vi "ReadtextandwriteSql.vi"() -> ()   [LabVIEW 2019]
uses:
  <vilib>/addons/database/Auxilliary.llb/DB Tools Parameter Info.ctl
  <vilib>/addons/database/Auxilliary.llb/DB Tools DataTypes.ctl
  <vilib>/addons/database/Auxilliary.llb/DB Tools Parameter Dir.ctl
  <vilib>/addons/database/Connection.llb/DB Tools Open Connec (String).vi
  <vilib>/Utility/file.llb/Read Delimited Spreadsheet (string).vi
  <vilib>/addons/database/Auxilliary.llb/DB Tools Format Datetime String (Time Stamp).vi
  <vilib>/addons/database/Command.llb/Cmd Set Parameter Value (C).vi
  <vilib>/addons/database/Command.llb/Cmd Execute.vi
  <vilib>/addons/database/Recordset.llb/Rec Destroy - Command.vi
  <vilib>/addons/database/Command.llb/Cmd Delete.vi
  <vilib>/addons/database/NI_Database_API.lvlib
panel:
  out "spreadsheet string":string
  out "insert time":timestamp
  out "total time in opreation":dbl
  out "Program start time":timestamp
  out "size(s)":i32[](array[numeric])
  out "Current Number of file":i32
  out "Current record number":i32
  out "all rows 2":string[](array[string])
  out "all rows":string[][](array[string])
  out "Total  Content Read from file":i32
  out "Content of Current file":string
  out "Current File path":path
  out "No of text files in folder":dbl
  in  "Input for folder path":path
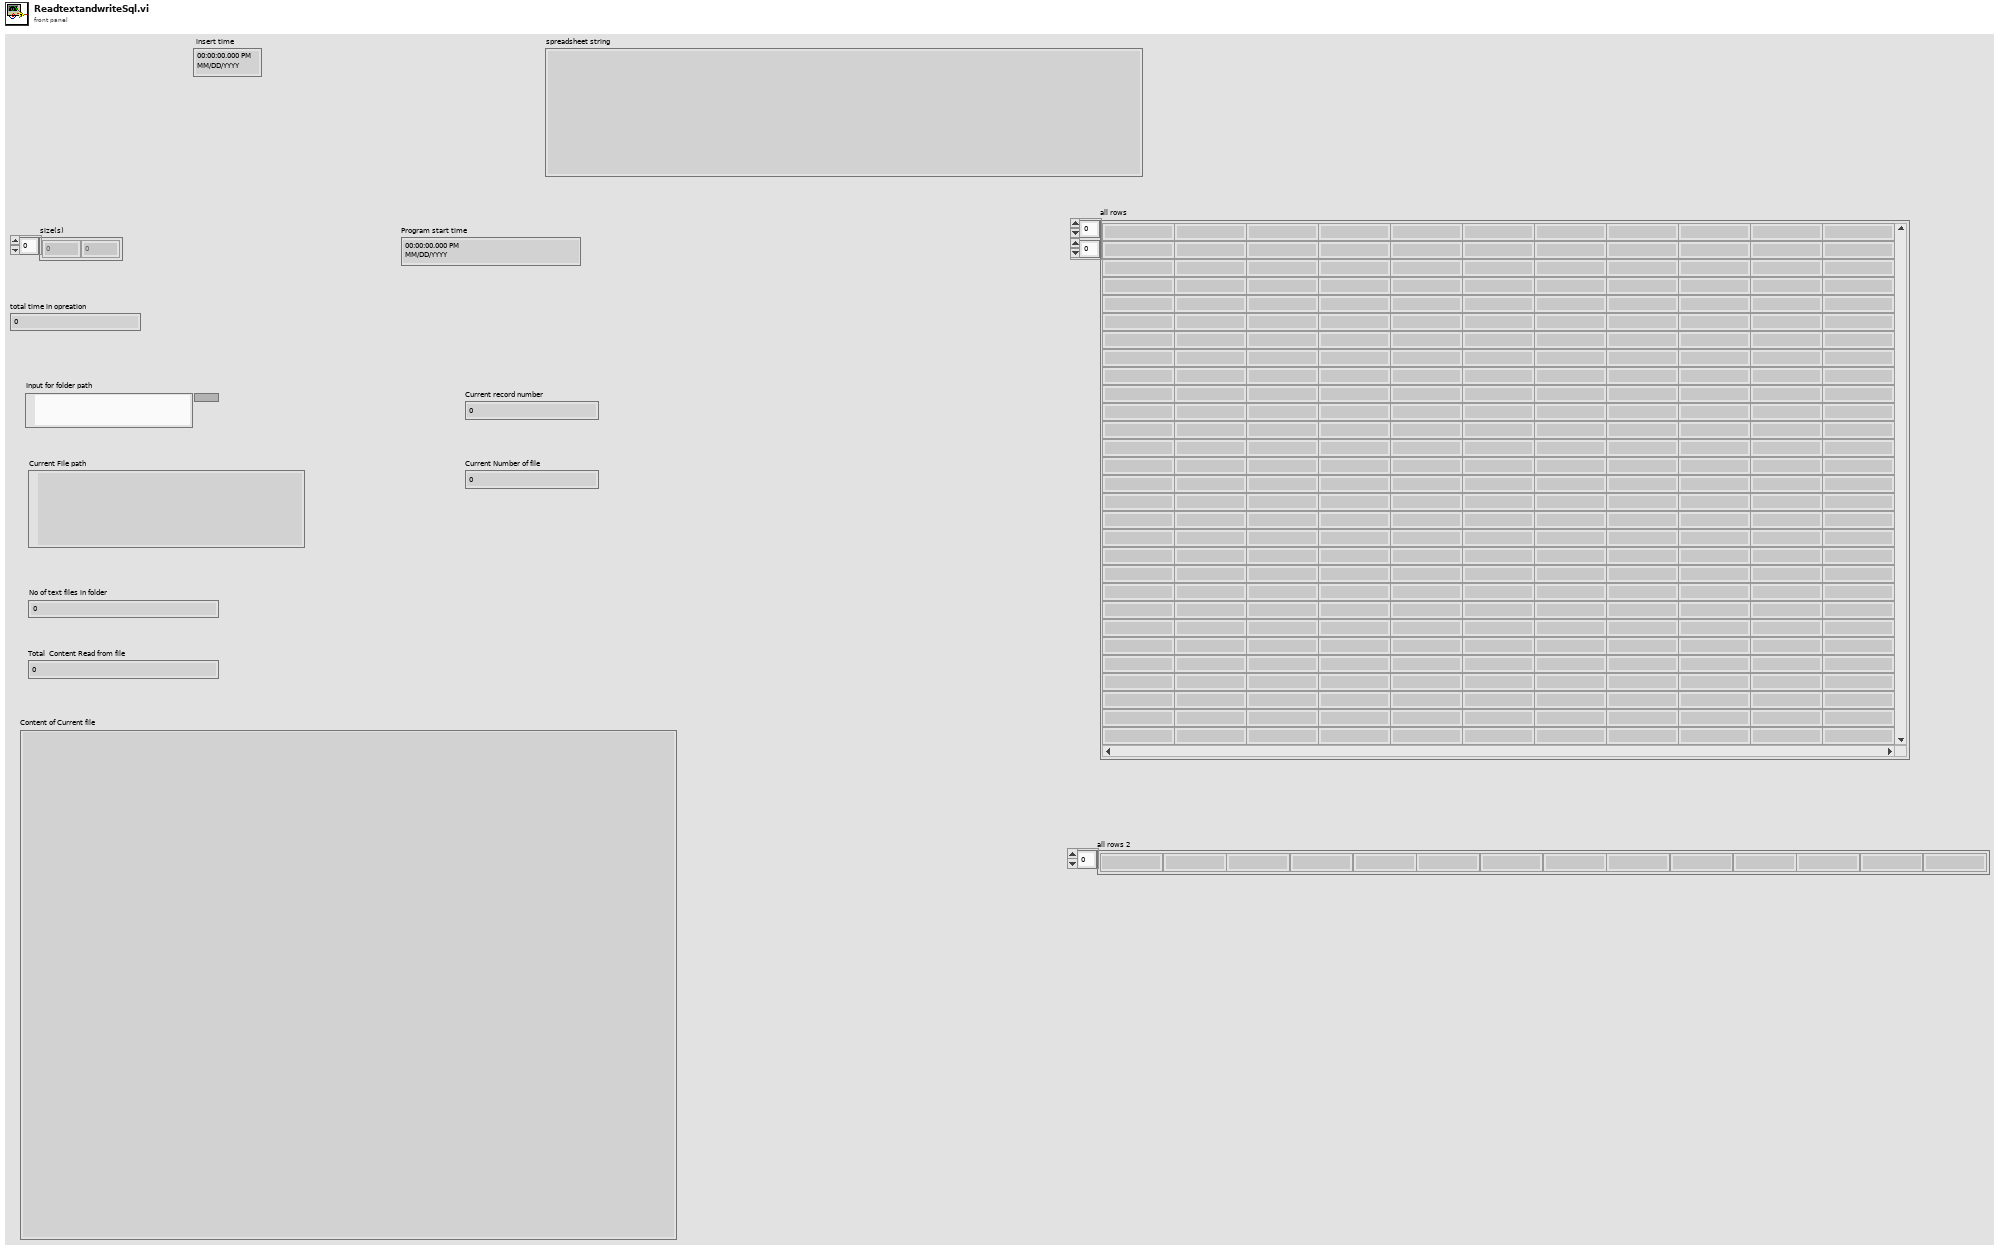
[diagram p1: front panel]
types:
  T1 = typedef "NI_Database_API.lvlib/DB Tools Parameter Info.ctl" = cluster{"parameter name":string, "type":T2, "direction":T3, "value":variant}
  T2 = typedef "NI_Database_API.lvlib/DB Tools DataTypes.ctl" = enum16{"String", "Long (I32)", "Single (SGL)", "Double (DBL)", "Date/Time", "Binary"}
  T3 = typedef "NI_Database_API.lvlib/DB Tools Parameter Dir.ctl" = enum32{"Input", "Output", "Input/Output", "Return Value"}
  T4 = typedef "NI_Database_API.lvlib/Conn ObjectReference.ctl" = refnum<k1>
  T5 = typedef "NI_Database_API.lvlib/Cmd ObjectReference.ctl" = refnum<k1>
  T6 = typedef "NI_Database_API.lvlib/Cmd-Rec Object Reference.ctl" = refnum<k1>
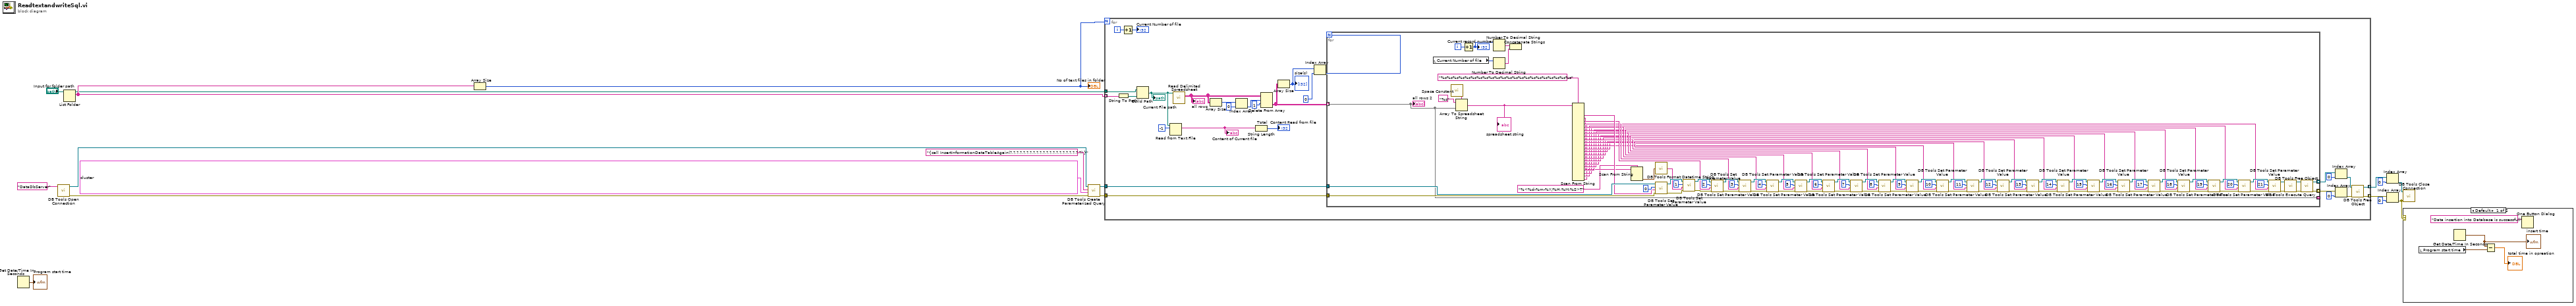
[diagram p0: block diagram]
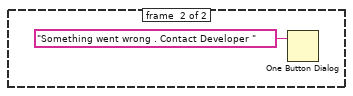
[diagram p2: hidden frame]
diagram:
  n1 = Get Date/Time In Seconds() -> (seconds since 1Jan1904=→"Program start time":timestamp)
  n2 = call-poly <vilib>:"DB Tools Open Connection.vi"("connection information"="DataDbServer") -> ("error out"=w13:errorcluster, "connection reference"=w12:T4)  [unwired: 7 in]
  n3 = List Folder(path="Input for folder path") -> (path out=w16:path, filenames=w17:string[])  [unwired: 3 in, 2 out]
  n4 = Array Size(array=w17) -> (size(s)=w14:i32)
  "No of text files in folder" <- w14
  n5 = call <vilib>:"DB Tools Create Parameterized Query.vi"("error in (no error)"=w13, "parameters"=T1[] [{"parameter name"="Start", "type"=enum."String", "direction"=enum."Input", "value"=variant}, {"parameter name"="DateTime", "type"=enum."Date/Time", "direction"=enum."Input", "value"=variant}, {"parameter name"="RollNo", "type"=enum."String", "direction"=enum."Input", "value"=variant}, {"parameter name"="Grade", "type"=enum."String", "direction"=enum."Input", "value"=variant}, {"parameter name"="BatchNO", "type"=enum."String", "direction"=enum."Input", "value"=variant}, {"parameter name"="product", "type"=enum."String", "direction"=enum."Input", "value"=variant}, {"parameter name"="OPName", "type"=enum."String", "direction"=enum."Input", "value"=variant}, {"parameter name"="shiftName", "type"=enum."String", "direction"=enum."Input", "value"=variant}, {"parameter name"="width", "type"=enum."String", "direction"=enum."Input", "value"=variant}, {"parameter name"="EWeight", "type"=enum."String", "direction"=enum."Input", "value"=variant}, {"parameter name"="TSetPoint", "type"=enum."String", "direction"=enum."Input", "value"=variant}, {"parameter name"="BSetPoint", "type"=enum."String", "direction"=enum."Input", "value"=variant}, {"parameter name"="col113", "type"=enum."String", "direction"=enum."Input", "value"=variant}, {"parameter name"="col14", "type"=enum."String", "direction"=enum."Input", "value"=variant}, {"parameter name"="col15", "type"=enum."String", "direction"=enum."Input", "value"=variant}, {"parameter name"="col16", "type"=enum."String", "direction"=enum."Input", "value"=variant}, {"parameter name"="col17", "type"=enum."String", "direction"=enum."Input", "value"=variant}, {"parameter name"="col18", "type"=enum."String", "direction"=enum."Input", "value"=variant}, {"parameter name"="col19", "type"=enum."String", "direction"=enum."Input", "value"=variant}, {"parameter name"="col20", "type"=enum."String", "direction"=enum."Input", "value"=variant}, {"parameter name"="col21", "type"=enum."String", "direction"=enum."Input", "value"=variant}, {"parameter name"="col22", "type"=enum."String", "direction"=enum."Input", "value"=variant}], "SQL query"="{call InsertInformationDataTableAgain(?,?,?,?,?,?,?,?,?,?,?,?,?,?,?,?,?,?,?,?,?,?) }", "connection reference"=w12) -> ("error out"=w8:errorcluster, "command reference"=w9:T5)  [unwired: 3 in, 1 out]
  n6 = for {
    N: w14 -> [_]
    tunnel: w17 -> [w46] mode=indexing
    tunnel: w16 -> [w45]
    tunnel: w9 -> [w34]
    tunnel: w8 -> [w33]
    tunnel: [w26] -> w7 mode=indexing
    tunnel: [w25] -> w5 mode=indexing
    i -> [w36]
    n7 = String To Path(string=w46) -> (path=w44:path)
    n8 = Increment(x=w36) -> (x+1=→"Current Number of file":i32)
    n9 = Build Path(base path=w45, name or relative path=w44) -> (appended path=w42:path)
    "Current File path" <- w42
    n10 = Read from Text File(file (use dialog)=w42, count=-1) -> (text=w41:string)  [unwired: 2 in, 3 out]
    "Content of Current file" <- w41
    n11 = call-poly <vilib>:"Read Delimited Spreadsheet.vi"("file path (dialog if empty)"=w42) -> ("all rows"=w20:string[][])  [unwired: 9 in, 5 out]
    "all rows" <- w20
    n12 = Array Size(array=w20) -> (size(s)=w24:i32[])
    n13 = Index Array(array=w24, index=0) -> (element=w22:i32)
    n14 = String Length(string=w41) -> (length=→"Total  Content Read from file":i32)
    n15 = Delete From Array(array=w20, length=w22, index (row)=1) -> (deleted portion=w19:string[][])  [unwired: 1 in, 1 out]
    n16 = Array Size(array=w19) -> (size(s)=w39:i32[])
    "size(s)" <- w39
    n17 = Index Array "Index Array"(array=w39, index=0) -> (element=w37:i32)
    n18 = for {
      N: w37 -> [_]
      tunnel: w19 -> [w51] mode=indexing
      tunnel: [w51] -> _ mode=indexing
      tunnel: w34 -> [w151]
      tunnel: w33 -> [w100]
      tunnel: [w78] -> w32 mode=indexing
      tunnel: [w77] -> w29 mode=indexing
      i -> [w103]
      n19 = local read "Current Number of file"() -> (w106:i32)
      n20 = call <vilib>:"Space Constant.vi"() -> ("String"=w50:string)
      n21 = Array To Spreadsheet String(delimiter (Tab)=w50, array=w51, 3:"%s" ("format string")) -> (spreadsheet string=w52:string)
      "spreadsheet string" <- w52
      n22 = Increment(x=w103) -> (x+1=w102:i32)
      "Current record number" <- w102
      n23 = Number To Decimal String(number=w102) -> (decimal integer string=w105:string)  [unwired: 1 in]
      n24 = Number To Decimal String(number=w106) -> (decimal integer string=w104:string)  [unwired: 1 in]
      n25 = Concatenate Strings(w105, w104) -> ()  [unwired: 1 out]
      n26 = Scan From String(format string="%s%s%s%s%s%s%s%s%s%s%s%s%s%s%s%s%s%s%s%s%s%s", input string=w52) -> (output 1=w74:string, output 2=w49:string, output 3=w73:string, output 4=w72:string, output 5=w71:string, output 6=w70:string, output 7=w69:string, output 8=w68:string, output 9=w67:string, output 10=w66:string, output 11=w65:string, output 12=w64:string, output 13=w63:string, output 14=w61:string, output 15=w60:string, output 16=w59:string, output 17=w58:string, output 18=w57:string, output 19=w56:string, output 20=w55:string, output 21=w54:string, output 22=w53:string)  [unwired: 24 in, 3 out]
      n27 = Scan From String(format string="%<%d-%m-%Y/%H:%M:%S>T", input string=w49) -> (output 1=w48:timestamp)  [unwired: 3 in, 3 out]
      n28 = call-poly <vilib>:"DB Tools Format Datetime String.vi"("time stamp"=w48) -> ("date/time string"=w75:string)
      n29 = call-poly <vilib>:"DB Tools Set Parameter Value.vi"("error in (no error)"=w100, "value"=w74, "parameter index"=0, "command reference"=w151) -> ("error out"=w101:errorcluster, "command reference out"=w149:T5)  [unwired: 4 in]
      n30 = call-poly <vilib>:"DB Tools Set Parameter Value.vi"("error in (no error)"=w101, "value"=w75, "parameter index"=1, "command reference"=w149) -> ("error out"=w147:errorcluster, "command reference out"=w146:T5)  [unwired: 4 in]
      n31 = call-poly <vilib>:"DB Tools Set Parameter Value.vi"("error in (no error)"=w147, "value"=w73, "parameter index"=2, "command reference"=w146) -> ("error out"=w143:errorcluster, "command reference out"=w144:T5)  [unwired: 4 in]
      n32 = call-poly <vilib>:"DB Tools Set Parameter Value.vi"("error in (no error)"=w143, "value"=w72, "parameter index"=3, "command reference"=w144) -> ("error out"=w98:errorcluster, "command reference out"=w141:T5)  [unwired: 4 in]
      n33 = call-poly <vilib>:"DB Tools Set Parameter Value.vi"("error in (no error)"=w98, "value"=w71, "parameter index"=4, "command reference"=w141) -> ("error out"=w139:errorcluster, "command reference out"=w140:T5)  [unwired: 4 in]
      n34 = call-poly <vilib>:"DB Tools Set Parameter Value.vi"("error in (no error)"=w139, "value"=w70, "parameter index"=5, "command reference"=w140) -> ("error out"=w136:errorcluster, "command reference out"=w137:T5)  [unwired: 4 in]
      n35 = call-poly <vilib>:"DB Tools Set Parameter Value.vi"("error in (no error)"=w136, "value"=w69, "parameter index"=6, "command reference"=w137) -> ("error out"=w133:errorcluster, "command reference out"=w134:T5)  [unwired: 4 in]
      n36 = call-poly <vilib>:"DB Tools Set Parameter Value.vi"("error in (no error)"=w133, "value"=w68, "parameter index"=7, "command reference"=w134) -> ("error out"=w130:errorcluster, "command reference out"=w131:T5)  [unwired: 4 in]
      n37 = call-poly <vilib>:"DB Tools Set Parameter Value.vi"("error in (no error)"=w130, "value"=w67, "parameter index"=8, "command reference"=w131) -> ("error out"=w127:errorcluster, "command reference out"=w128:T5)  [unwired: 4 in]
      n38 = call-poly <vilib>:"DB Tools Set Parameter Value.vi"("error in (no error)"=w127, "value"=w66, "parameter index"=9, "command reference"=w128) -> ("error out"=w124:errorcluster, "command reference out"=w125:T5)  [unwired: 4 in]
      n39 = call-poly <vilib>:"DB Tools Set Parameter Value.vi"("error in (no error)"=w124, "value"=w65, "parameter index"=10, "command reference"=w125) -> ("error out"=w122:errorcluster, "command reference out"=w121:T5)  [unwired: 4 in]
      n40 = call-poly <vilib>:"DB Tools Set Parameter Value.vi"("error in (no error)"=w122, "value"=w64, "parameter index"=11, "command reference"=w121) -> ("error out"=w119:errorcluster, "command reference out"=w120:T5)  [unwired: 4 in]
      n41 = call-poly <vilib>:"DB Tools Set Parameter Value.vi"("error in (no error)"=w119, "value"=w63, "parameter index"=12, "command reference"=w120) -> ("error out"=w62:errorcluster, "command reference out"=w117:T5)  [unwired: 4 in]
      n42 = call-poly <vilib>:"DB Tools Set Parameter Value.vi"("error in (no error)"=w62, "value"=w61, "parameter index"=13, "command reference"=w117) -> ("error out"=w115:errorcluster, "command reference out"=w114:T5)  [unwired: 4 in]
      n43 = call-poly <vilib>:"DB Tools Set Parameter Value.vi"("error in (no error)"=w115, "value"=w60, "parameter index"=14, "command reference"=w114) -> ("error out"=w111:errorcluster, "command reference out"=w112:T5)  [unwired: 4 in]
      n44 = call-poly <vilib>:"DB Tools Set Parameter Value.vi"("error in (no error)"=w111, "value"=w59, "parameter index"=15, "command reference"=w112) -> ("error out"=w108:errorcluster, "command reference out"=w109:T5)  [unwired: 4 in]
      n45 = call-poly <vilib>:"DB Tools Set Parameter Value.vi"("error in (no error)"=w108, "value"=w58, "parameter index"=16, "command reference"=w109) -> ("error out"=w96:errorcluster, "command reference out"=w95:T5)  [unwired: 4 in]
      n46 = call-poly <vilib>:"DB Tools Set Parameter Value.vi"("error in (no error)"=w96, "value"=w57, "parameter index"=17, "command reference"=w95) -> ("error out"=w92:errorcluster, "command reference out"=w93:T5)  [unwired: 4 in]
      n47 = call-poly <vilib>:"DB Tools Set Parameter Value.vi"("error in (no error)"=w92, "value"=w56, "parameter index"=18, "command reference"=w93) -> ("error out"=w89:errorcluster, "command reference out"=w90:T5)  [unwired: 4 in]
      n48 = call-poly <vilib>:"DB Tools Set Parameter Value.vi"("error in (no error)"=w89, "value"=w55, "parameter index"=19, "command reference"=w90) -> ("error out"=w87:errorcluster, "command reference out"=w86:T5)  [unwired: 4 in]
      n49 = call-poly <vilib>:"DB Tools Set Parameter Value.vi"("error in (no error)"=w87, "value"=w54, "parameter index"=20, "command reference"=w86) -> ("error out"=w83:errorcluster, "command reference out"=w84:T5)  [unwired: 4 in]
      n50 = call-poly <vilib>:"DB Tools Set Parameter Value.vi"("error in (no error)"=w83, "value"=w53, "parameter index"=21, "command reference"=w84) -> ("error out"=w81:errorcluster, "command reference out"=w82:T5)  [unwired: 4 in]
      n51 = call-poly <vilib>:"DB Tools Execute Query.vi"("error in (no error)"=w81, "command reference"=w82) -> ("error out"=w80:errorcluster, "command-recordset reference"=w79:T6)  [unwired: 6 in]
      n52 = call-poly <vilib>:"DB Tools Free Object.vi"("error in (no error)"=w80, "command-recordset reference"=w79) -> ("error out"=w77:errorcluster, "command reference"=w78:T5)  [unwired: 8 in]
      "all rows 2" <- w51
    }
    n53 = Index Array(array=w32, index=0) -> (element=w30:T5)
    n54 = Index Array(array=w29, index=0) -> (element=w27:errorcluster)
    n55 = call-poly <vilib>:"DB Tools Free Object.vi"("error in (no error)"=w27, "command reference"=w30) -> ("error out"=w25:errorcluster, "connection reference"=w26:T4)  [unwired: 8 in]
  }
  n56 = Index Array(array=w7, index=0) -> (element=w3:T4)
  n57 = Index Array(array=w5, index=0) -> (element=w2:errorcluster)
  n58 = call <vilib>:"DB Tools Close Connection.vi"("error in (no error)"=w2, "connection reference"=w3) -> ()  [unwired: 5 in, 1 out]
  n59 = case shown="Default" w2 {
    frame #0 {
      n60 = local read "Program start time"() -> (w155:timestamp)
      n61 = Get Date/Time In Seconds() -> (seconds since 1Jan1904=w156:timestamp)
      "insert time" <- w156
      n62 = Subtract(x=w156, y=w155) -> (x-y=→"total time in opreation":dbl)
      n63 = One Button Dialog(message="Data insertion into Database is successfull") -> ()  [unwired: 1 in, 1 out]
    }
    frame #1 {
      n64 = One Button Dialog(message="Something went wrong . Contact Developer ") -> ()  [unwired: 1 in, 1 out]
    }
  }
